vi "FPGA Test Harness.vi"() -> ()   [LabVIEW 2018]
uses:
  <vilib>/FPGAPlugInAG/cRIO-9056/niLvFpga_Open_cRIO-9056.vi
  <vilib>/FPGAPlugInAG/cRIO-9056/niLvFpga_Run_cRIO-9056.vi
  <vilib>/Utility/error.llb/Error Cluster From Error Code.vi
  <vilib>/rvi/errors/niLvFpgaAdjustHostInterfaceError.vi
  <vilib>/FPGAPlugInAG/cRIO-9056/niLvFpga_Close_cRIO-9056.vi
  <vilib>/rvi/interface/nirviOpenFPGA/nirviOpenFPGA.xnode
  FPGA Bitfiles/NewCompressorRig_CompressorFPGA_FPGAMain_lmgdCTsM3i0.lvbitx
  FPGA/FPGA Main.vi
  <vilib>/rvi/interface/nirviMethod/nirviMethod.xnode
  <vilib>/rvi/interface/nirviReadWriteControl/nirviReadWriteControl.xnode
  <vilib>/LabVIEW Targets/FPGA/cRIO/shared/nicrio_ModuleControls/nicrio_cRIO-9237_DataRatesRing.ctl
  <vilib>/rvi/interface/nirviCloseFPGA/nirviCloseFPGA.xnode
  <vilib>/rvi/errors/niLvFpgaMergeErrorWithErrorCode.vi
  NiFpgaLv.dll
  <vilib>/FPGAPlugInAG/cRIO-9056/niLvFpga_ReadFifo_cRIO-9056.vi
  <vilib>/FPGAPlugInAG/cRIO-9056/niLvFpga_StartFifo_cRIO-9056.vi
  <vilib>/FPGAPlugInAG/cRIO-9056/niLvFpga_StopFifo_cRIO-9056.vi
panel:
  in  "Quit":bool
  in  "Stream":bool
  out "Old":sgl[](array[numeric])
  out "New":sgl[](array[numeric])
  out "Safe Voltage":fxp<+/-,20,5>[](array[numeric])
  out "Voltage Out":fxp<+/-,20,5>[](array[numeric])
  out "Safe":bool[](array[boolean])
  out "Mod 8":bool[](array[boolean])
  out "Mod 7":bool[](array[boolean])
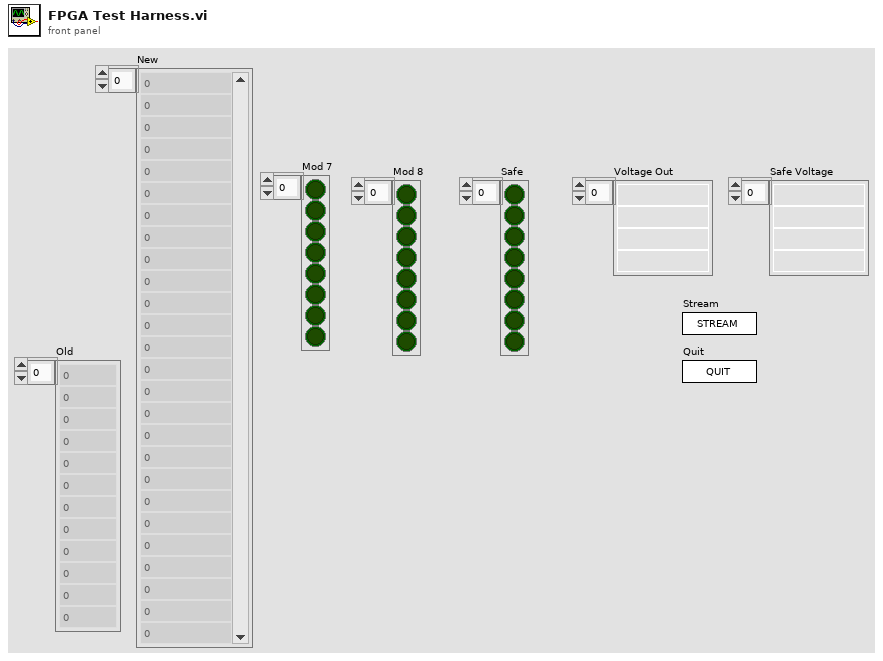
[diagram p1: front panel]
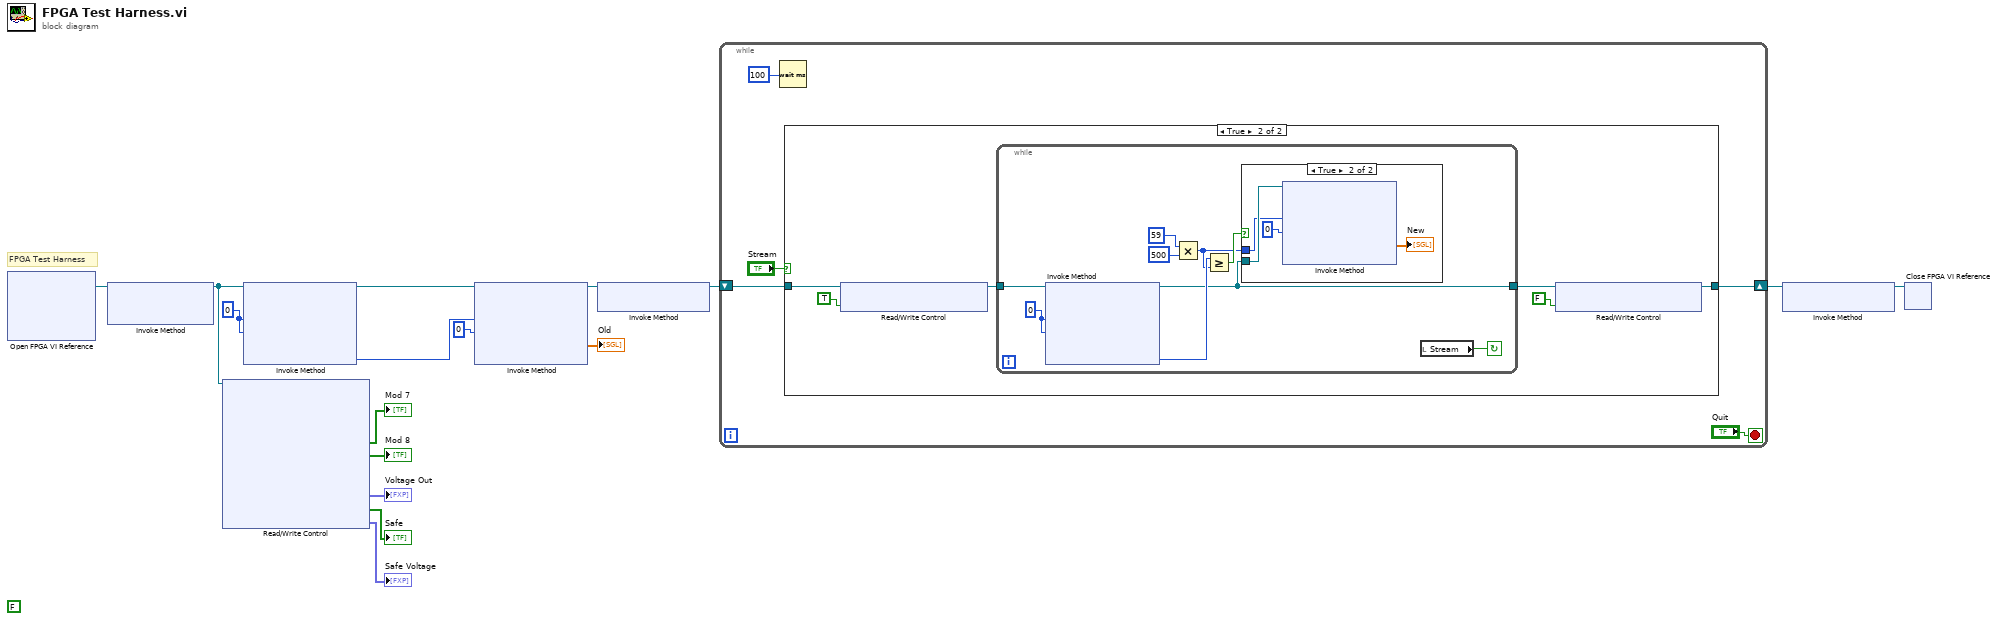
[diagram p0: block diagram]
diagram:
  (unwired) FALSE ("STOP")
  w9 = u32 0 ("Number of Elements")
  # "FPGA Test Harness"
  n1 = xnode "Open FPGA VI Reference"() -> ("FPGA VI Reference Out"=w11:refnum<k20>)  [unwired: 2 in, 1 out]
  n2 = xnode "Invoke Method"("FPGA VI Reference In"=w11) -> ("FPGA VI Reference Out"=w5:refnum<k20>)  [unwired: 2 in, 1 out]
  n3 = xnode "Read/Write Control"("FPGA VI Reference In"=w5) -> ("Mod 7"=→"Mod 7":bool[], "Mod 8"=→"Mod 8":bool[], "Voltage Out"=→"Voltage Out":fxp<+/-,20,5>[], "Safe Digital"=→"Safe":bool[], "Safe Voltage"=→"Safe Voltage":fxp<+/-,20,5>[])  [unwired: 1 in, 7 out]
  n4 = xnode "Invoke Method"("FPGA VI Reference In"=w5, "Number of Elements"=w9, "Timeout (ms)"=w9) -> ("FPGA VI Reference Out"=w10:refnum<k20>, "Elements Remaining"=w8:u32)  [unwired: 1 in, 2 out]
  n5 = xnode "Invoke Method"("FPGA VI Reference In"=w10, "Number of Elements"=w8, "Timeout (ms)"=0) -> ("FPGA VI Reference Out"=w6:refnum<k20>, "Data"=→"Old":sgl[])  [unwired: 1 in, 2 out]
  n6 = xnode "Invoke Method"("FPGA VI Reference In"=w6) -> ("FPGA VI Reference Out"=w2:refnum<k20>)  [unwired: 1 in, 1 out]
  n7 = while {
    shift-right: [w17] -> w1
    shift-left: w2 -> [w18]
    stop <- "Quit" stop-if-true
    n8 = Wait (ms)(milliseconds to wait=u32 100) -> ()  [unwired: 1 out]
    n9 = case shown="True" "Stream" {
      tunnel: w18 -> [w22 w28]
      tunnel: [w22 w23] -> w17
      frame False {
      }
      frame True {
        n10 = xnode "Read/Write Control"("FPGA VI Reference In"=w28, "Analogue stream"=TRUE) -> ("FPGA VI Reference Out"=w26:refnum<k20>)  [unwired: 1 in, 1 out]
        n11 = while {
          tunnel: w26 -> [w37]
          tunnel: [w30] -> w25
          stop <- w29 continue-if-true
          w36 = u32 0 ("Number of Elements")
          n12 = xnode "Invoke Method"("FPGA VI Reference In"=w37, "Number of Elements"=w36, "Timeout (ms)"=w36) -> ("FPGA VI Reference Out"=w30:refnum<k20>, "Elements Remaining"=w35:u32)  [unwired: 1 in, 2 out]
          n13 = Multiply(x=u32 59 ("y"), y=u32 500) -> (x*y=w31:u32)
          n14 = Greater Or Equal?(x=w35, y=w31) -> (x >= y?=w32:bool)
          n15 = case shown="True" w32 {
            tunnel: w30 -> [_ w40]
            tunnel: w31 -> [_ w39]
            frame False {
            }
            frame True {
              n16 = xnode "Invoke Method"("FPGA VI Reference In"=w40, "Number of Elements"=w39, "Timeout (ms)"=0) -> ("Data"=→"New":sgl[])  [unwired: 1 in, 3 out]
            }
          }
          n17 = local read "Stream"() -> (w29:bool)
        }
        n18 = xnode "Read/Write Control"("FPGA VI Reference In"=w25, "Analogue stream"=FALSE) -> ("FPGA VI Reference Out"=w23:refnum<k20>)  [unwired: 1 in, 1 out]
      }
    }
  }
  n19 = xnode "Invoke Method"("FPGA VI Reference In"=w1) -> ("FPGA VI Reference Out"=w3:refnum<k20>)  [unwired: 1 in, 1 out]
  n20 = xnode "Close FPGA VI Reference"("FPGA VI Reference In"=w3) -> ()  [unwired: 1 in, 1 out]
